vi "Logging Equals - Entries.vi"(1 "Entries A":T1[](array[typedef]), 2 "Entries B":T1[](array[typedef])) -> (5 "Equal":bool)   [LabVIEW 2012, in "femtoRoboLib.lvlib"]
uses:
  femtoRoboLib.lvlib
  Controls/Log Entry.ctl
  Controls/Log Value Type.ctl
  Controls/Log Value Cluster.ctl
  Logging Equals - Entry.vi
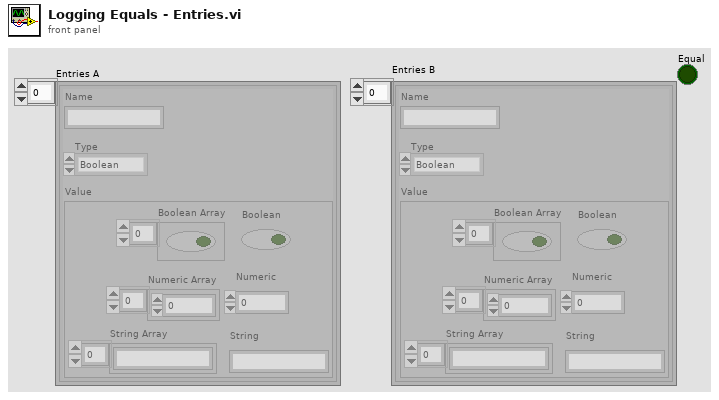
[diagram p1: front panel]
types:
  T1 = typedef "femtoRoboLib.lvlib/Log Entry.ctl" = cluster{"Name":string, "Type":T2, "Value":T3}
  T2 = typedef "femtoRoboLib.lvlib/Log Value Type.ctl" = enum16{"Boolean", "Numeric", "String", "Boolean Array", "Numeric Array", "String Array"}
  T3 = typedef "femtoRoboLib.lvlib/Log Value Cluster.ctl" = cluster{"Boolean Array":bool[], "Boolean":bool, "Numeric Array":dbl[], "Numeric":dbl, "String Array":string[], "String":string}
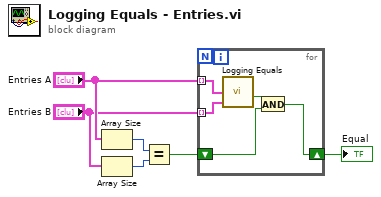
[diagram p0: block diagram]
diagram:
  n1 = Array Size(array="Entries A") -> (size(s)=w2:i32)
  n2 = Array Size(array="Entries B") -> (size(s)=w1:i32)
  n3 = Equal?(x=w2, y=w1) -> (x = y?=w3:bool)
  n4 = for {
    tunnel: "Entries A" -> [w9] mode=indexing
    tunnel: "Entries B" -> [w8] mode=indexing
    shift-right: [w11] -> w6
    shift-left: w3 -> [w10]
    n5 = call-poly "Logging Equals.vi"("Entry A"=w9, "Entry B"=w8) -> ("Equal"=w7:bool)  [unwired: 4 in]
    n6 = And(x=w7, y=w10) -> (x .and. y?=w11:bool)
  }
  "Equal" <- w6
